vi "SSL Referee Command to GUI Command.vi"(11 "stage":u64) -> (3 "String":string)   [LabVIEW 2016]
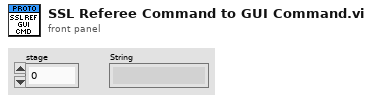
[diagram p1: front panel]
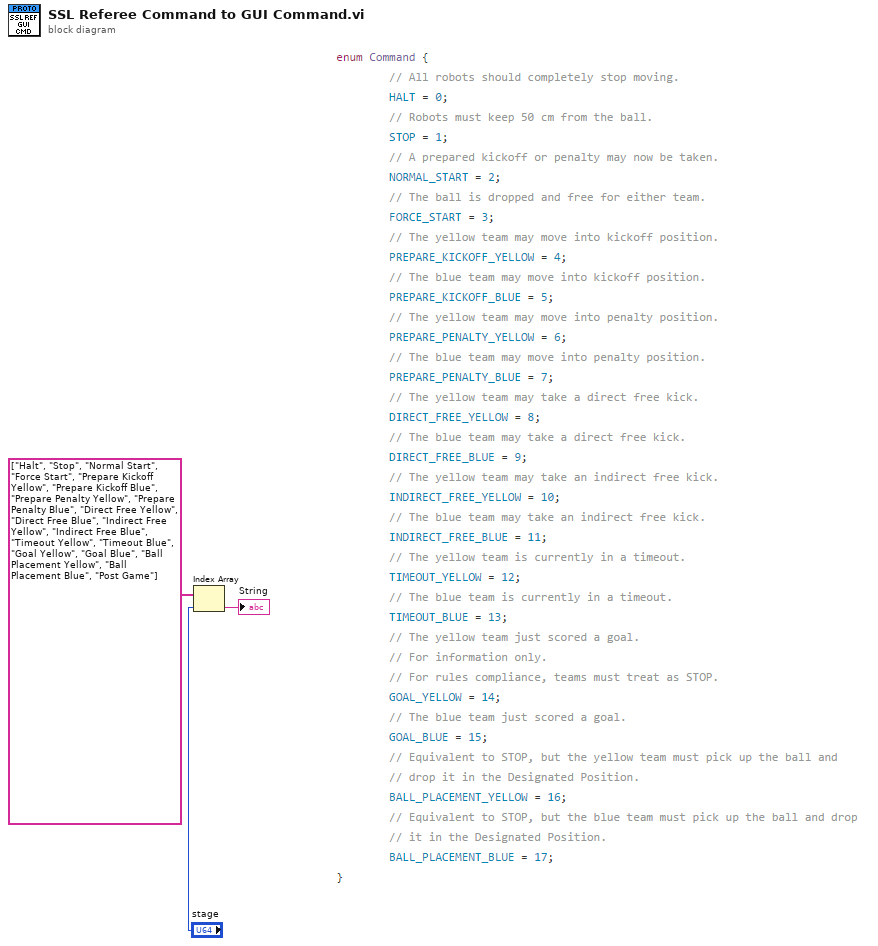
[diagram p0: block diagram]
diagram:
  n1 = Index Array(array=string[] ["Halt", "Stop", "Normal Start", "Force Start", "Prepare Kickoff Yellow", "Prepare Kickoff Blue", "Prepare Penalty Yellow", "Prepare Penalty Blue", "Direct Free Yellow", "Direct Free Blue", "Indirect Free Yellow", "Indirect Free Blue", "Timeout Yellow", "Timeout Blue", "Goal Yellow", "Goal Blue", "Ball Placement Yellow", "Ball Placement Blue", "Post Game"], index="stage") -> (element=→"String":string)
